vi "GAS_LEAK_SAFETY_INTERLOCK.vi"(1 "%LEL":dbl, 2 "%LEL Set-point":dbl) -> (0 "Alarm":bool)   [LabVIEW 2014]
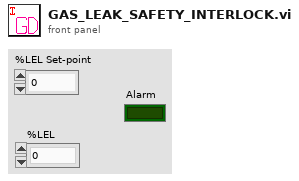
[diagram p1: front panel]
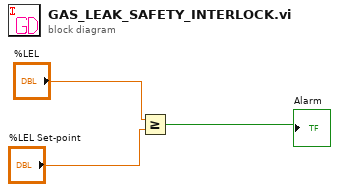
[diagram p0: block diagram]
diagram:
  n1 = Greater Or Equal?(x="%LEL", y="%LEL Set-point") -> (x >= y?=→"Alarm":bool)
